vi "Thingworx_RemoveQuotes.vi"(1 "Incoming string in":string) -> (0 "Incoming string out":string)   [LabVIEW 2016]
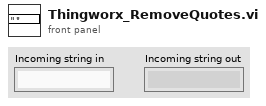
[diagram p1: front panel]
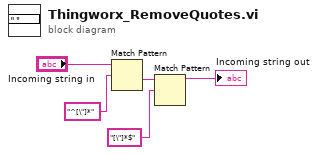
[diagram p0: block diagram]
diagram:
  n1 = Match Pattern(string="Incoming string in", regular expression="^[\"]*") -> (after substring=w4:string)  [unwired: 1 in, 3 out]
  n2 = Match Pattern(string=w4, regular expression="[\"]*$") -> (before substring=→"Incoming string out":string)  [unwired: 1 in, 3 out]
